vi "Teleop.vi"(0 "Call Context":T10) -> (6 "SubState 3":T4, 8 "SubState 4":T4, 9 "SubState 5":T9, 11 "Loop 3 Data":T5, 13 "Loop 4 Data":T3, 14 "SubState 0":T4=enum."driver control", 15 "Loop 1 Data":T7, 16 "Loop 0 Data":T8, 17 "SubState 1":T4, 18 "Loop 2 Data":T6, 19 "SubState 2":T4)   [LabVIEW 2012]
uses:
  typedefs/subStates.ctl
  <vilib>/Rock Robotics/WPI/DriverStation/WPI_DriverStationDerivedRobotMode.ctl
  typedefs/singleUseSubstate.ctl
  typedefs/Loop Datatypes/Loop 0 Datatype.ctl
  typedefs/Loop Datatypes/Loop 1 Datatype.ctl
  typedefs/Loop Datatypes/Loop 2 Datatype.ctl
  typedefs/Loop Datatypes/Loop 3 Datatype.ctl
  typedefs/Loop Datatypes/Loop 4 Datatype.ctl
  <vilib>/Rock Robotics/WPI/Joystick/WPI_JoystickDevRef.ctl
  <vilib>/Rock Robotics/WPI/Joystick/WPI_JoystickDeviceEnum.ctl
  typedefs/fg_typedef.ctl
  <vilib>/Rock Robotics/WPI/Joystick/WPI_JoystickGetSetRefNum.vi
panel:
  out "Drive to DC":bool
  out "JS2 Button 9":bool
  out "JS3":T1
  out "JS1":T1
  out "JS2":T1
  out "Exit Value":i32=-1
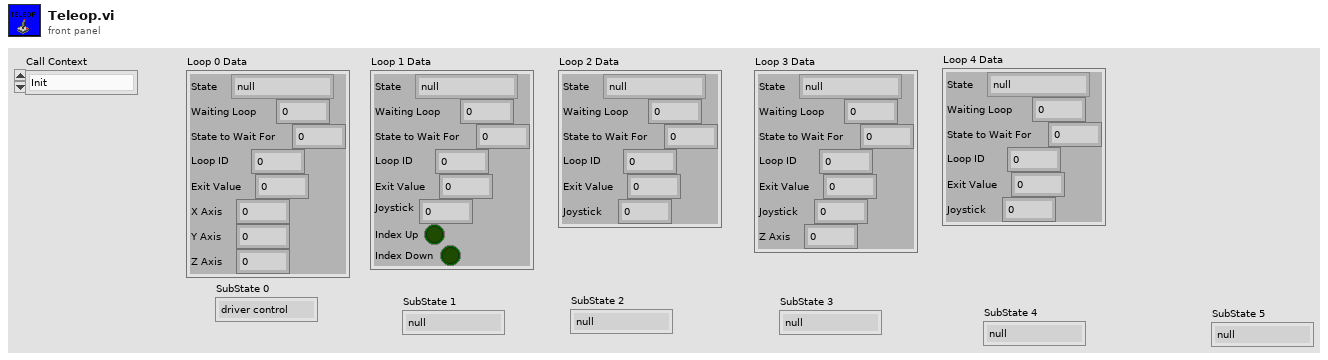
[diagram p1: front panel]
types:
  T1 = typedef "WPI_JoystickDevRef.ctl" = cluster{"Device":T2}
  T2 = typedef "WPI_JoystickDeviceEnum.ctl" = enum16{"USB 1", "USB 2", "USB 3", "USB 4", "Kinect 1", "Kinect 2"}
  T3 = typedef "Loop 4 Datatype.ctl" = cluster{"State":T4, "Waiting Loop":i32, "State to Wait For":i32, "Loop ID":i32, "Exit Value":i32, "Joystick":dbl}
  T4 = typedef "subStates.ctl" = enum16{"null", "wait", "driver control", "auto", "manual override", "hold position", "rotate", "feeder", "end"}
  T5 = typedef "Loop 3 Datatype.ctl" = cluster{"State":T4, "Waiting Loop":i32, "State to Wait For":i32, "Loop ID":i32, "Exit Value":i32, "Joystick":dbl, "Z Axis":dbl}
  T6 = typedef "Loop 2 Datatype.ctl" = cluster{"State":T4, "Waiting Loop":i32, "State to Wait For":i32, "Loop ID":i32, "Exit Value":i32, "Joystick":dbl}
  T7 = typedef "Loop 1 Datatype.ctl" = cluster{"State":T4, "Waiting Loop":i32, "State to Wait For":i32, "Loop ID":i32, "Exit Value":i32, "Joystick":dbl, "Index Up":bool, "Index Down":bool}
  T8 = typedef "Loop 0 Datatype.ctl" = cluster{"State":T4, "Waiting Loop":i32, "State to Wait For":i32, "Loop ID":i32, "Exit Value":i32, "X Axis":dbl, "Y Axis":dbl, "Z Axis":dbl}
  T9 = typedef "singleUseSubstate.ctl" = enum16{"null", "wait", "shift high", "shift low"}
  T10 = typedef "WPI_DriverStationDerivedRobotMode.ctl" = enum16{"Init", "Execute", "Stop"}
  T11 = cluster{"axis 1 (x)":dbl, "axis 2 (y)":dbl, "axis 3 (throttle)":dbl, "axis 4":dbl, "axis 5":dbl, "axis 6":dbl}
  T12 = typedef "WPI_JoystickButtonState.ctl" = cluster{"Button 1":bool, "Button 2":bool, "Button 3":bool, "Button 4":bool, "Button 5":bool, "Button 6":bool, "Button 7":bool, "Button 8":bool, "Button 9":bool, "Button 10":bool, "Button 11":bool, "Button 12":bool}
  T13 = typedef "fg_typedef.ctl" = enum16{"Get", "Set"}
  T14 = typedef "WPI_EncoderDevRef.ctl" = cluster{"DevStatus":errorcluster, "EncoderIndex":T15, "CounterIndex":T16, "DistancePerCount":dbl, "Decoding Type":T17}
  T15 = typedef "FPGA_EncoderIdx.ctl" = enum8{"Enc 0", "Enc 1", "Enc 2", "Enc 3", "Invalid"}
  T16 = typedef "FPGA_CounterCtrSystemIndex.ctl" = enum8{"Ctr 0", "Ctr 1", "Ctr 2", "Ctr 3", "Ctr 4", "Ctr 5", "Ctr 6", "Ctr 7", "Invalid"}
  T17 = typedef "WPI_EncoderType.ctl" = enum16{"1x", "2x", "4x"}
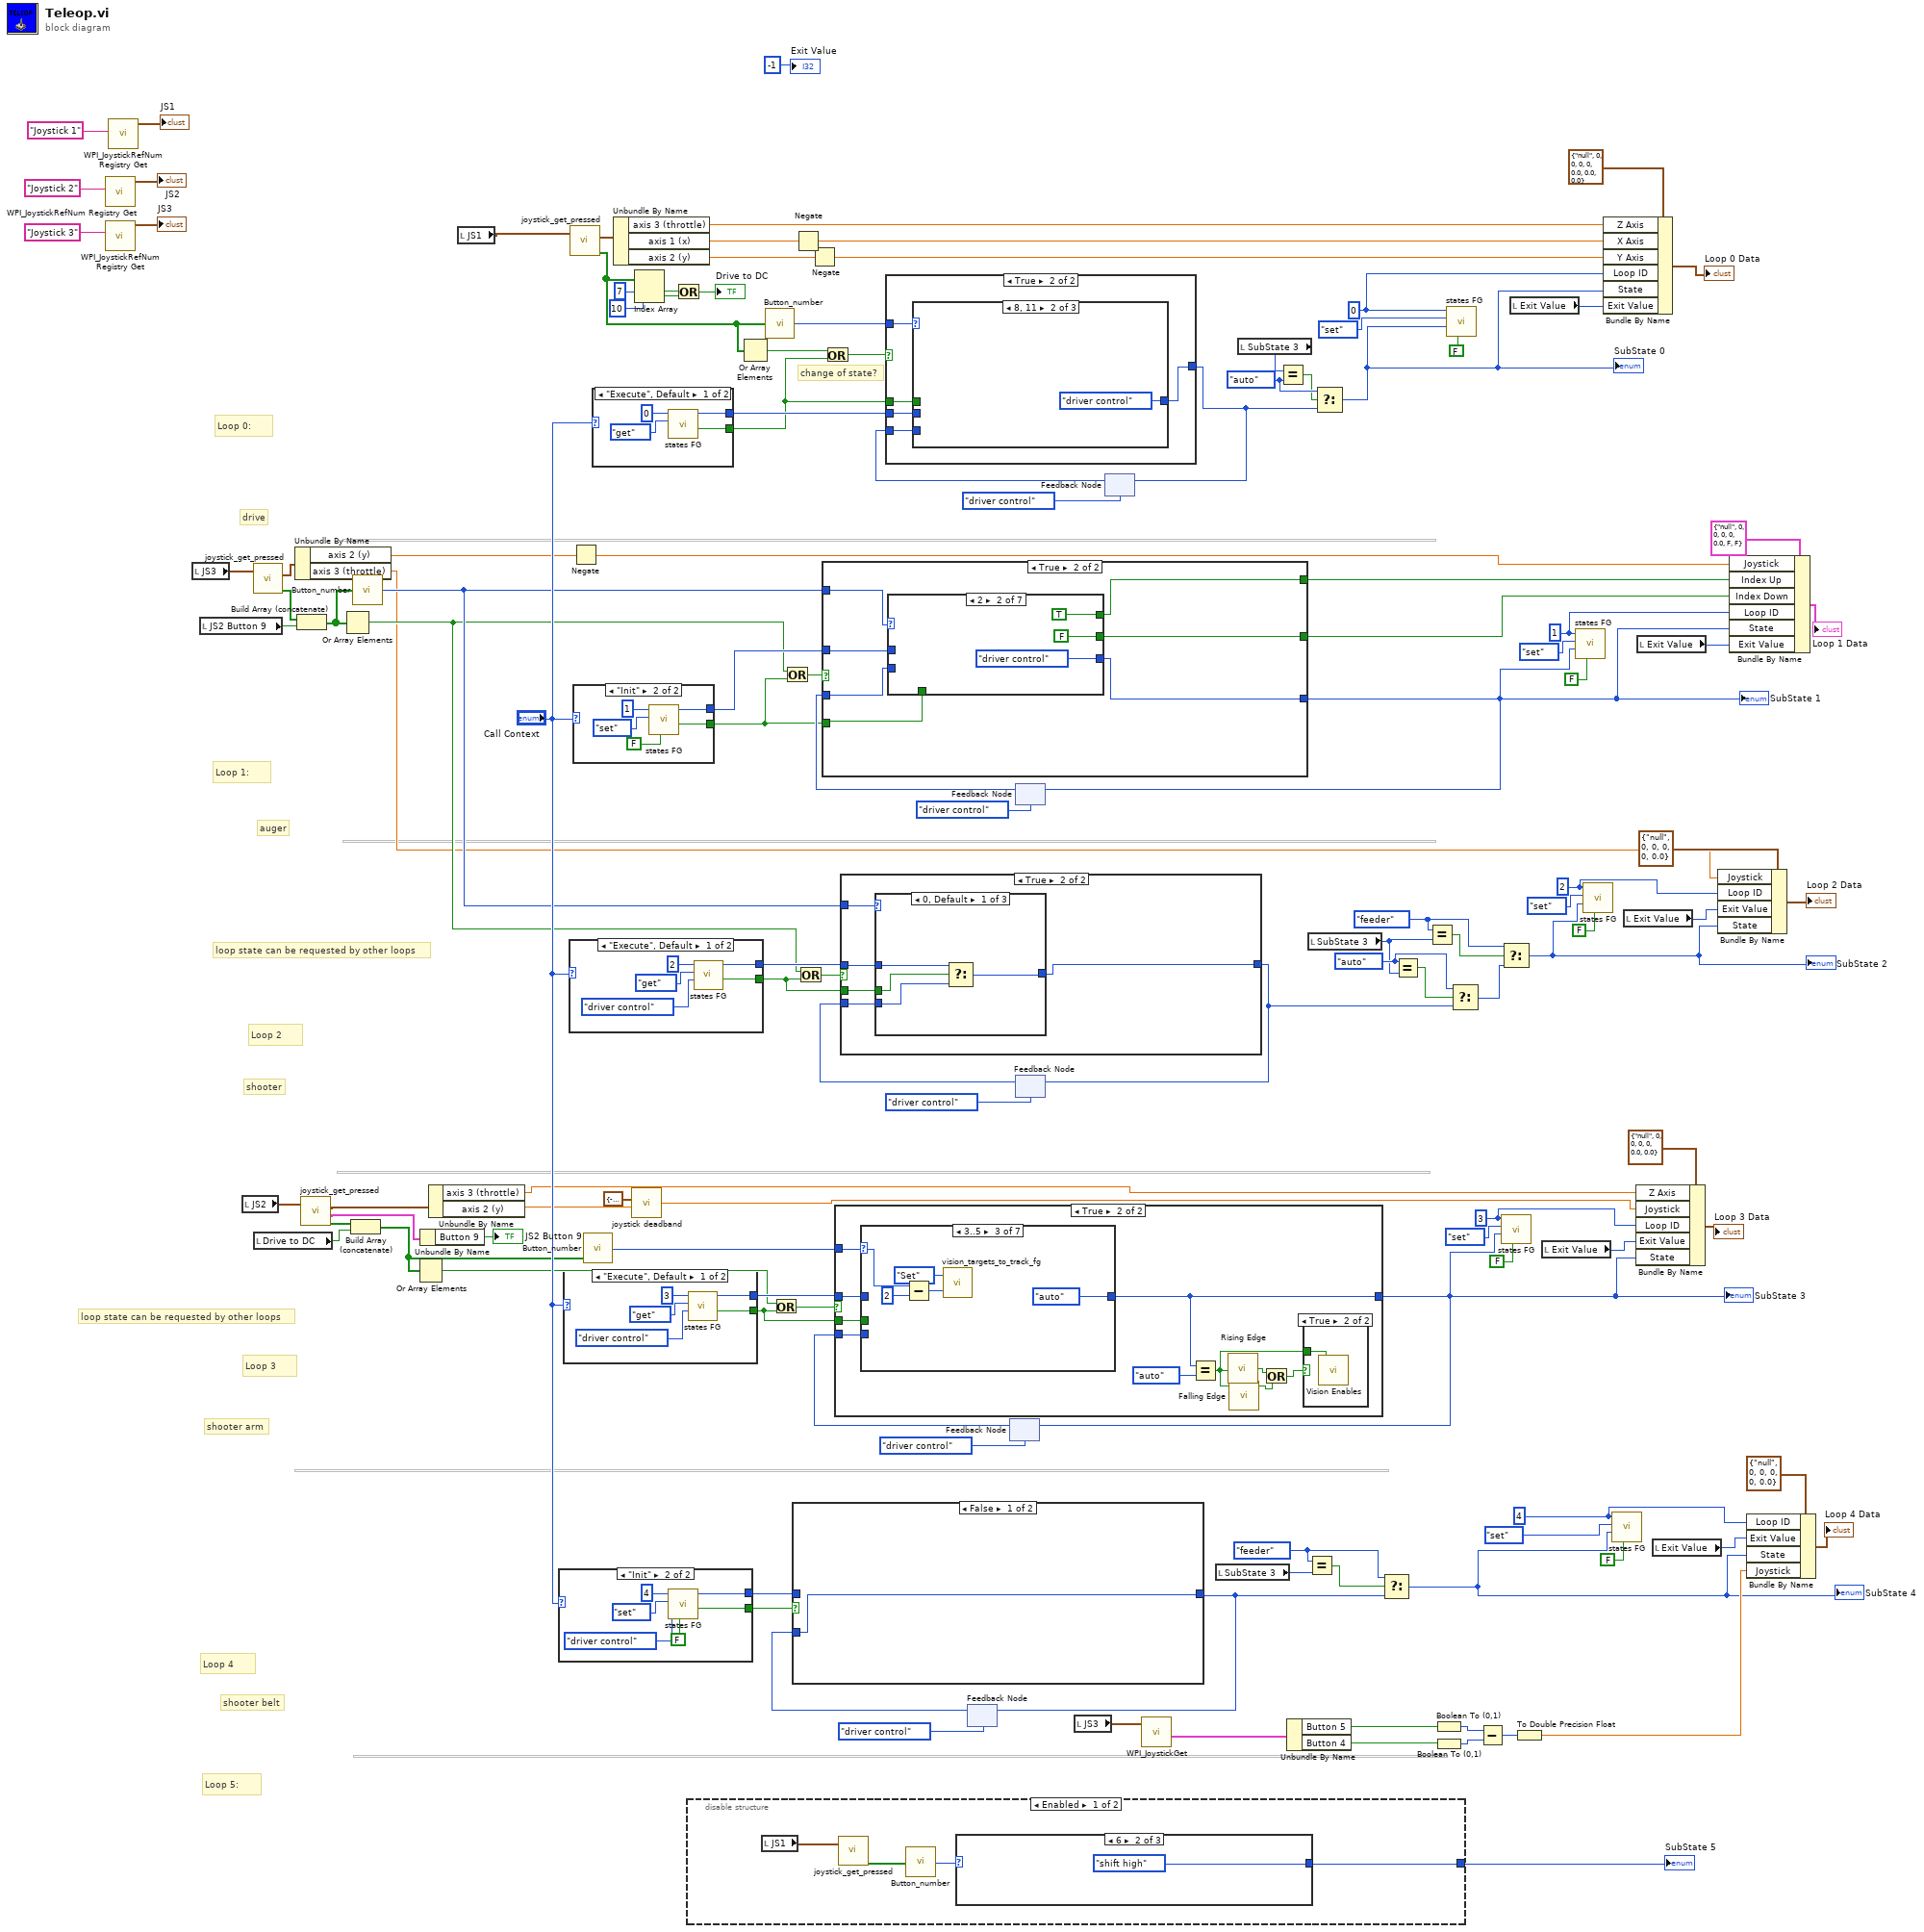
[diagram p0: block diagram]
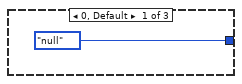
[diagram p2: hidden frame]
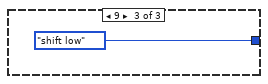
[diagram p3: hidden frame]
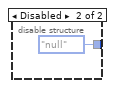
[diagram p4: hidden frame]
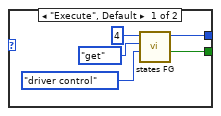
[diagram p6: hidden frame]
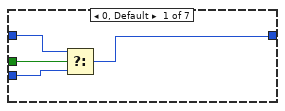
[diagram p9: hidden frame]
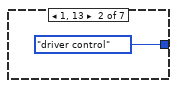
[diagram p10: hidden frame]
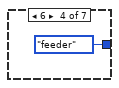
[diagram p11: hidden frame]
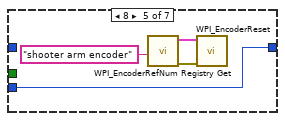
[diagram p12: hidden frame]
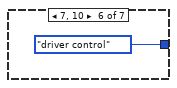
[diagram p13: hidden frame]
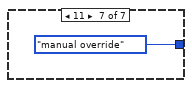
[diagram p14: hidden frame]
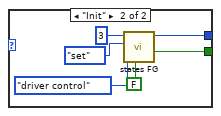
[diagram p15: hidden frame]
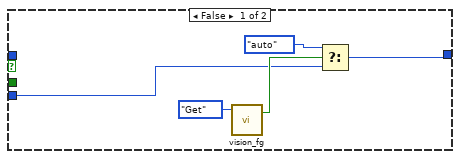
[diagram p16: hidden frame]
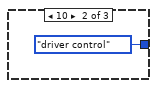
[diagram p17: hidden frame]
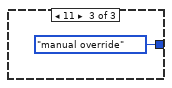
[diagram p18: hidden frame]
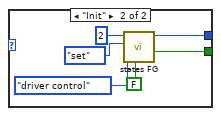
[diagram p19: hidden frame]
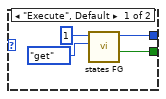
[diagram p20: hidden frame]
diagram:
  w20 = subStates."auto" ("y")
  w23 = subStates."auto" ("x")
  w30 = subStates."feeder" ("x")
  w32 = subStates."feeder" ("x")
  w88 = 4 ("Loop ID")
  w103 = 3 ("Loop ID")
  w104 = 2 ("Loop ID")
  w113 = 1 ("Loop ID")
  w115 = 0 ("Loop ID")
  # "shooter belt"
  # "shooter arm"
  # "Loop 4"
  # "Loop 3"
  # "loop state can be requested by other loops"
  # "drive"
  # "auger"
  # "shooter"
  # "change of state?"
  # "Loop 5:"
  # "Loop 2"
  # "Loop 1:"
  # "Loop 0:"
  # "loop state can be requested by other loops"
  n1 = call <vilib>:"WPI_JoystickRefNum Registry Get.vi"("refnum name"="Joystick 2") -> ("JoystickDevRef"=→"JS2":T1)  [unwired: 9 in, 1 out]
  n2 = call <vilib>:"WPI_JoystickRefNum Registry Get.vi"("refnum name"="Joystick 3") -> ("JoystickDevRef"=→"JS3":T1)  [unwired: 9 in, 1 out]
  n3 = call <vilib>:"WPI_JoystickRefNum Registry Get.vi"("refnum name"="Joystick 1") -> ("JoystickDevRef"=→"JS1":T1)  [unwired: 9 in, 1 out]
  n4 = local read "JS3"() -> (w67:T1)
  n5 = local read "JS2 Button 9"() -> (w51:bool)
  n6 = local read "JS2"() -> (w43:T1)
  n7 = call "joystick_get_pressed.vi"("JoystickDevRef 2"=w67) -> ("Axes"=w66:T11, "Buttons Pressed?"=w26:bool[])  [unwired: 1 in, 2 out]
  n8 = local read "Drive to DC"() -> (w3:bool)
  n9 = Unbundle By Name(w66) -> ("axis 2 (y)"=w75:dbl, "axis 3 (throttle)"=w53:dbl)
  n10 = Build Array (concatenate)(w26, w51) -> (w25:bool[])
  n11 = call "joystick_get_pressed.vi"("JoystickDevRef 2"=w43) -> ("Axes"=w49:T11, "Buttons"=w48:T12, "Buttons Pressed?"=w46:bool[])  [unwired: 1 in, 1 out]
  n12 = Or Array Elements(Boolean array=w25) -> (logical OR=w55:bool)
  n13 = Build Array (concatenate)(w46, w3) -> (w4:bool[])
  n14 = call "Button_number.vi"("Button Array"=w25) -> ("Button Pressed"=w57:i32)
  n15 = Or Array Elements(Boolean array=w4) -> (logical OR=w47:bool)
  n16 = Unbundle By Name(w48) -> ("Button 9"=→"JS2 Button 9":bool)
  n17 = Unbundle By Name(w49) -> ("axis 3 (throttle)"=w12:dbl, "axis 2 (y)"=w16:dbl)
  n18 = local read "JS1"() -> (w68:T1)
  n19 = case shown="\"Init\"" "Call Context" {
    tunnel: [w134 w140] -> w40
    tunnel: [w132 w137] -> w90
    frame "Execute", Default {
      n20 = call "states FG.vi"("subState in"=subStates."driver control", "menu (get)"=enum16{"set", "get"}."get", "Loop ID"=4) -> ("exit out"=w134:bool, "subState out"=w132:T4)  [unwired: 5 in, 2 out]
    }
    frame "Init" {
      n21 = call "states FG.vi"("exit in"=FALSE, "subState in"=subStates."driver control", "menu (get)"=enum16{"set", "get"}."set", "Loop ID"=4) -> ("exit out"=w140:bool, "subState out"=w137:T4)  [unwired: 4 in, 2 out]
    }
  }
  n22 = case shown="\"Execute\", Default" "Call Context" {
    tunnel: [w145 w151] -> w44
    tunnel: [w143 w148] -> w101
    frame "Execute", Default {
      n23 = call "states FG.vi"("subState in"=subStates."driver control", "menu (get)"=enum16{"set", "get"}."get", "Loop ID"=3) -> ("exit out"=w145:bool, "subState out"=w143:T4)  [unwired: 5 in, 2 out]
    }
    frame "Init" {
      n24 = call "states FG.vi"("exit in"=FALSE, "subState in"=subStates."driver control", "menu (get)"=enum16{"set", "get"}."set", "Loop ID"=3) -> ("exit out"=w151:bool, "subState out"=w148:T4)  [unwired: 4 in, 2 out]
    }
  }
  n25 = case shown="\"Execute\", Default" "Call Context" {
    tunnel: [w156 w162] -> w54
    tunnel: [w154 w159] -> w120
    frame "Execute", Default {
      n26 = call "states FG.vi"("subState in"=subStates."driver control", "menu (get)"=enum16{"set", "get"}."get", "Loop ID"=2) -> ("exit out"=w156:bool, "subState out"=w154:T4)  [unwired: 5 in, 2 out]
    }
    frame "Init" {
      n27 = call "states FG.vi"("exit in"=FALSE, "subState in"=subStates."driver control", "menu (get)"=enum16{"set", "get"}."set", "Loop ID"=2) -> ("exit out"=w162:bool, "subState out"=w159:T4)  [unwired: 4 in, 2 out]
    }
  }
  n28 = call "joystick_get_pressed.vi"("JoystickDevRef 2"=w68) -> ("Axes"=w74:T11, "Buttons Pressed?"=w10:bool[])  [unwired: 1 in, 2 out]
  n29 = Negate(x=w75) -> (-x=w60:dbl)
  n30 = case shown="\"Init\"" "Call Context" {
    tunnel: [w166 w171] -> w61
    tunnel: [w165 w169] -> w117
    frame "Execute", Default {
      n31 = call "states FG.vi"("menu (get)"=enum16{"set", "get"}."get", "Loop ID"=1) -> ("exit out"=w166:bool, "subState out"=w165:T4)  [unwired: 6 in, 2 out]
    }
    frame "Init" {
      n32 = call "states FG.vi"("exit in"=FALSE, "menu (get)"=enum16{"set", "get"}."set", "Loop ID"=1) -> ("exit out"=w171:bool, "subState out"=w169:T4)  [unwired: 5 in, 2 out]
    }
  }
  n33 = call "Button_number.vi"("Button Array"=w4) -> ("Button Pressed"=w45:i32)
  n34 = case shown="\"Execute\", Default" "Call Context" {
    tunnel: [w175 w180] -> w64
    tunnel: [w174 w178] -> w118
    frame "Execute", Default {
      n35 = call "states FG.vi"("menu (get)"=enum16{"set", "get"}."get", "Loop ID"=0) -> ("exit out"=w175:bool, "subState out"=w174:T4)  [unwired: 6 in, 2 out]
    }
    frame "Init" {
      n36 = call "states FG.vi"("exit in"=FALSE, "menu (get)"=enum16{"set", "get"}."set", "Loop ID"=0) -> ("exit out"=w180:bool, "subState out"=w178:T4)  [unwired: 5 in, 2 out]
    }
  }
  n37 = Unbundle By Name(w74) -> ("axis 3 (throttle)"=w11:dbl, "axis 1 (x)"=w81:dbl, "axis 2 (y)"=w80:dbl)
  n38 = call "joystick deadband.vi"("Joystick In"=w16, "Deadband Range"=cluster{"Deadband Min":dbl, "Deadband Max":dbl} {"Deadband Min"=-0.05, "Deadband Max"=0.05}) -> ("Joystick Out"=w15:dbl)  [unwired: 4 in]
  n39 = Index Array(array=w10, index #1=7 ("index"), index #2=10 ("index")) -> (element #1=w7:bool, element #2=w6:bool)
  n40 = Or(x=w7, y=w6) -> (x .or. y?=→"Drive to DC":bool)
  n41 = disable-structure shown="Enabled" {
    disable-tunnel: [w184 singleUseSubstate."null" ("SubState 5")] -> w84
    frame Enabled {
      n42 = local read "JS1"() -> (w183:T1)
      n43 = call "joystick_get_pressed.vi"("JoystickDevRef 2"=w183) -> ("Buttons Pressed?"=w186:bool[])  [unwired: 1 in, 3 out]
      n44 = call "Button_number.vi"("Button Array"=w186) -> ("Button Pressed"=w185:i32)
      n45 = case shown="6" w185 {
        tunnel: [singleUseSubstate."null" ("Enum") singleUseSubstate."shift high" ("Enum") singleUseSubstate."shift low" ("Enum")] -> w184
        frame 0, Default {
        }
        frame 6 {
        }
        frame 9 {
        }
      }
    }
    frame Disabled {
    }
  }
  "SubState 5" <- w84
  n46 = Or Array Elements(Boolean array=w10) -> (logical OR=w65:bool)
  n47 = call "Button_number.vi"("Button Array"=w10) -> ("Button Pressed"=w73:i32)
  n48 = Or(x=w47, y=w44) -> (x .or. y?=w50:bool)
  n49 = Or(x=w55, y=w61) -> (x .or. y?=w62:bool)
  n50 = Negate(x=w81) -> (-x=w79:dbl)
  n51 = Or(x=w55, y=w54) -> (x .or. y?=w56:bool)
  n52 = Negate(x=w80) -> (-x=w78:dbl)
  n53 = Or(x=w65, y=w64) -> (x .or. y?=w63:bool)
  n54 = feedback #1(subStates."driver control" ("Drive SubState")) -> (w93:T4)
  n55 = case shown="False" w40 {
    tunnel: w93 -> [w191 _]
    tunnel: [w191 w192] -> w27
    tunnel: w90 -> [_ w192]
    frame False {
    }
    frame True {
    }
  }
  n56 = feedback-in #1(w27) -> ()
  n57 = feedback #2(subStates."driver control" ("Drive SubState")) -> (w98:T4)
  n58 = case shown="True" w50 {
    tunnel: w98 -> [w193 w198]
    tunnel: [w193 w199] -> w76
    tunnel: w101 -> [_ w201]
    tunnel: w45 -> [_ w203]
    tunnel: w44 -> [_ w202]
    frame False {
    }
    frame True {
      n59 = case shown="3..5" w203 {
        selector: w203 -> [_ _ w212 _ _ _ _]
        tunnel: w202 -> [w208 _ _ _ _ _ _]
        tunnel: w198 -> [w207 _ _ _ w216 _ _]
        tunnel: w201 -> [w206 _ _ _ _ _ _]
        tunnel: [w205 subStates."driver control" ("Drive SubState") subStates."auto" ("Drive SubState") subStates."feeder" ("Drive SubState") w216 subStates."driver control" ("Drive SubState") subStates."manual override" ("Drive SubState")] -> w199
        frame 0, Default {
          n60 = Select(t=w206, s=w208, f=w207) -> (s? t:f=w205:T4)
        }
        frame 1, 13 {
        }
        frame 3..5 {
          n61 = Subtract(x=w212, y=2) -> (x-y=w210:i32)
          n62 = call "vision_targets_to_track_fg.vi"("Input"=w210, "Menu (Get)"=fg_typedef."Set") -> ()  [unwired: 1 out]
        }
        frame 6 {
        }
        frame 8 {
          n63 = call <vilib>:"WPI_EncoderRefNum Registry Get.vi"("refnum name"="shooter arm encoder") -> ("error out"=w218:errorcluster, "EncoderDevRef"=w217:T14)  [unwired: 9 in]
          n64 = call <vilib>:"WPI_EncoderReset.vi"("error in (no error)"=w218, "EncoderDevRef"=w217) -> ()  [unwired: 8 in, 2 out]
        }
        frame 7, 10 {
        }
        frame 11 {
        }
      }
      n65 = Equal?(x=w199, y=subStates."auto") -> (x = y?=w194:bool)
      n66 = call "Rising Edge.vi"("Input"=w194) -> ("Rising Edge"=w197:bool)
      n67 = call "Falling Edge.vi"("Input"=w194) -> ("Output"=w196:bool)  [unwired: 4 in]
      n68 = Or(x=w197, y=w196) -> (x .or. y?=w195:bool)
      n69 = case shown="True" w195 {
        tunnel: w194 -> [_ w204]
        frame False {
        }
        frame True {
          n70 = call "Vision Enables.vi"("enable/disable"=w204) -> ()  [unwired: 1 in]
        }
      }
    }
  }
  "SubState 3" <- w76
  n71 = feedback-in #2(w76) -> ()
  n72 = feedback #3(subStates."driver control" ("Drive SubState")) -> (w119:T4)
  n73 = case shown="True" w62 {
    tunnel: w119 -> [w222 w228]
    tunnel: [w222 w223] -> w77
    tunnel: w117 -> [_ w229]
    tunnel: w57 -> [_ w227]
    tunnel: w61 -> [_ w226]
    tunnel: [_ w225] -> w59
    tunnel: [_ w224] -> w58
    frame False {
    }
    frame True {
      n74 = case shown="2" w227 {
        tunnel: w229 -> [w233 _ _ _ _ _ _]
        tunnel: w228 -> [w232 _ _ _ _ _ w251]
        tunnel: [w231 subStates."driver control" ("Drive SubState") subStates."driver control" ("Drive SubState") subStates."driver control" ("Drive SubState") subStates."manual override" ("Drive SubState") subStates."driver control" ("Drive SubState") w251] -> w223
        tunnel: w226 -> [w234 _ _ _ _ _ _]
        tunnel: [w230 TRUE FALSE w241 w243 w245 w247] -> w225
        tunnel: [w230 FALSE TRUE w241 w243 w245 w247] -> w224
        frame 0, Default {
          w230 = FALSE
          n75 = Select(t=w233, s=w234, f=w232) -> (s? t:f=w231:T4)
        }
        frame 2 {
        }
        frame 3 {
        }
        frame 6 {
          w241 = FALSE
        }
        frame 9 {
          w243 = FALSE
        }
        frame 8, 10 {
          w245 = FALSE
        }
        frame 13 {
          w247 = FALSE
          n76 = call <vilib>:"WPI_EncoderRefNum Registry Get.vi"("refnum name"="auger encoder") -> ("error out"=w249:errorcluster, "EncoderDevRef"=w248:T14)  [unwired: 9 in]
          n77 = call <vilib>:"WPI_EncoderReset.vi"("error in (no error)"=w249, "EncoderDevRef"=w248) -> ()  [unwired: 8 in, 2 out]
        }
      }
    }
  }
  "SubState 1" <- w77
  n78 = feedback-in #3(w77) -> ()
  n79 = feedback #4(subStates."driver control" ("Drive SubState")) -> (w123:T4)
  n80 = case shown="True" w56 {
    tunnel: w123 -> [w252 w258]
    tunnel: [w253 w257] -> w1
    tunnel: w120 -> [_ w259]
    tunnel: w57 -> [_ w261]
    tunnel: w54 -> [_ w260]
    frame False {
      n81 = call "vision_fg.vi"("Menu"=fg_typedef."Get") -> ("Enabled?"=w255:bool)  [unwired: 2 in, 1 out]
      n82 = Select(t=subStates."auto", s=w255, f=w252) -> (s? t:f=w253:T4)
    }
    frame True {
      n83 = case shown="0, Default" w261 {
        tunnel: w260 -> [w265 _ _]
        tunnel: w259 -> [w264 _ _]
        tunnel: w258 -> [w263 _ _]
        tunnel: [w262 subStates."driver control" ("Drive SubState") subStates."manual override" ("Drive SubState")] -> w257
        frame 0, Default {
          n84 = Select(t=w264, s=w265, f=w263) -> (s? t:f=w262:T4)
        }
        frame 10 {
        }
        frame 11 {
        }
      }
    }
  }
  n85 = feedback-in #4(w1) -> ()
  n86 = local read "JS3"() -> (w42:T1)
  n87 = feedback #5(subStates."driver control" ("Drive SubState")) -> (w125:T4)
  n88 = case shown="True" w63 {
    tunnel: w125 -> [w268 w270]
    tunnel: [w268 w269] -> w13
    tunnel: w118 -> [_ w271]
    tunnel: w73 -> [_ w273]
    tunnel: w64 -> [_ w272]
    frame False {
      # "keep current state, no change necessary"
    }
    frame True {
      n89 = case shown="8, 11" w273 {
        tunnel: w272 -> [w277 _ _]
        tunnel: w271 -> [w276 _ _]
        tunnel: w270 -> [w275 _ w283]
        tunnel: [w274 subStates."driver control" ("Drive SubState") w279] -> w269
        frame 0, Default {
          n90 = Select(t=w276, s=w277, f=w275) -> (s? t:f=w274:T4)
        }
        frame 8, 11 {
        }
        frame 7 {
          w280 = subStates."hold position" ("x")
          # "button 7, hold position toggle"
          n91 = Equal?(x=w280, y=w283) -> (x = y?=w282:bool)
          n92 = Select(t=subStates."driver control" ("Drive SubState"), s=w282, f=w280) -> (s? t:f=w279:T4)
        }
      }
    }
  }
  n93 = feedback-in #5(w13) -> ()
  n94 = call <vilib>:"WPI_JoystickGet.vi"("JoystickDevRef"=w42) -> ("Buttons"=w41:T12)  [unwired: 4 in, 2 out]
  n95 = local read "SubState 3"() -> (w29:T4)
  n96 = local read "SubState 3"() -> (w18:T4)
  n97 = Equal?(x=w18, y=w20) -> (x = y?=w19:bool)
  n98 = Unbundle By Name(w41) -> ("Button 5"=w39:bool, "Button 4"=w38:bool)
  n99 = local read "SubState 3"() -> (w21:T4)
  n100 = Equal?(x=w30, y=w29) -> (x = y?=w31:bool)
  n101 = Select(t=w20, s=w19, f=w13) -> (s? t:f=w17:T4)
  "SubState 0" <- w17
  n102 = Select(t=w30, s=w31, f=w27) -> (s? t:f=w28:T4)
  "SubState 4" <- w28
  n103 = Equal?(x=w23, y=w21) -> (x = y?=w24:bool)
  n104 = Equal?(x=w32, y=w21) -> (x = y?=w33:bool)
  n105 = Boolean To (0,1)(Boolean=w39) -> (0, 1=w36:i16)
  n106 = Boolean To (0,1)(Boolean=w38) -> (0, 1=w37:i16)
  n107 = call "states FG.vi"("exit in"=FALSE, "subState in"=w17, "menu (get)"=enum16{"set", "get"}."set", "Loop ID"=w115) -> ()  [unwired: 4 in, 4 out]
  n108 = Select(t=w23, s=w24, f=w1) -> (s? t:f=w22:T4)
  n109 = Subtract(x=w36, y=w37) -> (x-y=w35:i16)
  n110 = Select(t=w32, s=w33, f=w22) -> (s? t:f=w2:T4)
  "SubState 2" <- w2
  n111 = call "states FG.vi"("exit in"=FALSE, "subState in"=w76, "menu (get)"=enum16{"set", "get"}."set", "Loop ID"=w103) -> ()  [unwired: 4 in, 4 out]
  n112 = local read "Exit Value"() -> (w111:i32)
  n113 = To Double Precision Float(number=w35) -> (double precision float=w34:dbl)
  n114 = local read "Exit Value"() -> (w102:i32)
  n115 = call "states FG.vi"("exit in"=FALSE, "subState in"=w77, "menu (get)"=enum16{"set", "get"}."set", "Loop ID"=w113) -> ()  [unwired: 4 in, 4 out]
  n116 = call "states FG.vi"("exit in"=FALSE, "subState in"=w2, "menu (get)"=enum16{"set", "get"}."set", "Loop ID"=w104) -> ()  [unwired: 4 in, 4 out]
  n117 = Bundle By Name(cluster=T8 {"State"=enum."null", "Waiting Loop"=0, "State to Wait For"=0, "Loop ID"=0, "Exit Value"=0, "X Axis"=0.0, "Y Axis"=0.0, "Z Axis"=0.0} ("Cluster"), "Z Axis"=w11, "X Axis"=w79, "Y Axis"=w78, "Loop ID"=w115, "State"=w17, "Exit Value"=w111) -> (→"Loop 0 Data":T8)
  n118 = call "states FG.vi"("exit in"=FALSE, "subState in"=w28, "menu (get)"=enum16{"set", "get"}."set", "Loop ID"=w88) -> ()  [unwired: 4 in, 4 out]
  n119 = local read "Exit Value"() -> (w105:i32)
  n120 = Bundle By Name(cluster=T5 {"State"=enum."null", "Waiting Loop"=0, "State to Wait For"=0, "Loop ID"=0, "Exit Value"=0, "Joystick"=0.0, "Z Axis"=0.0} ("Loop 3 Data"), "Z Axis"=w12, "Joystick"=w15, "Loop ID"=w103, "Exit Value"=w102, "State"=w76) -> (→"Loop 3 Data":T5)
  n121 = local read "Exit Value"() -> (w110:i32)
  n122 = local read "Exit Value"() -> (w89:i32)
  n123 = Bundle By Name(cluster=T6 {"State"=enum."null", "Waiting Loop"=0, "State to Wait For"=0, "Loop ID"=0, "Exit Value"=0, "Joystick"=0.0} ("Loop 2 Data"), "Joystick"=w53, "Loop ID"=w104, "Exit Value"=w105, "State"=w2) -> (→"Loop 2 Data":T6)
  n124 = Bundle By Name(cluster=T7 {"State"=enum."null", "Waiting Loop"=0, "State to Wait For"=0, "Loop ID"=0, "Exit Value"=0, "Joystick"=0.0, "Index Up"=FALSE, "Index Down"=FALSE} ("Cluster"), "Joystick"=w60, "Index Up"=w59, "Index Down"=w58, "Loop ID"=w113, "State"=w77, "Exit Value"=w110) -> (→"Loop 1 Data":T7)
  n125 = Bundle By Name(cluster=T3 {"State"=enum."null", "Waiting Loop"=0, "State to Wait For"=0, "Loop ID"=0, "Exit Value"=0, "Joystick"=0.0} ("Loop 4 Data"), "Loop ID"=w88, "Exit Value"=w89, "State"=w28, "Joystick"=w34) -> (→"Loop 4 Data":T3)
  "Exit Value" <- -1 ("Exit Value")
